vi "Next.vi"(7 "Address":string, 8 "Error In":errorcluster) -> (0 "Error Out":errorcluster)   [LabVIEW 2018, in "Tests.lvlib" / "Known Hosts.lvlib"]
uses:
  Known Hosts.lvlib
  src/Toolkit/Known Hosts/Type Definitions/Get Results.ctl
  <vilib>/Utility/error.llb/Clear Errors.vi
  src/Toolkit/Known Hosts/Support/Create from Session.vi
  <vilib>/Utility/sysdir.llb/Get System Directory.vi
  src/Toolkit/Known Host/Support/Create from Known Hosts.vi
  src/Toolkit/Known Host/Support/Destroy to Known Hosts.vi
  src/Toolkit/Known Hosts/Support/Destroy to Session.vi
  <vilib>/addons/_JKI Toolkits/Caraya/classes/Test/Test.lvclass
  <vilib>/addons/_JKI Toolkits/Caraya/classes/Assert/Assert.lvclass
  src/Toolkit/Known Hosts/Known Hosts.lvclass
  Tests.lvlib
  src/Toolkit/Session/Session.lvclass
  src/Toolkit/Known Host/Known Host.lvclass
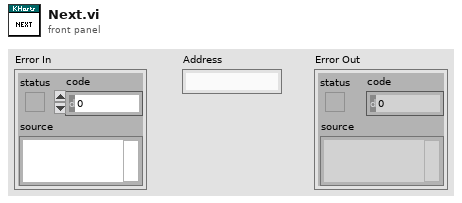
[diagram p1: front panel]
types:
  T1 = typedef "Toolkit.lvlib/Known Hosts.lvclass/Get Results.ctl" = i32
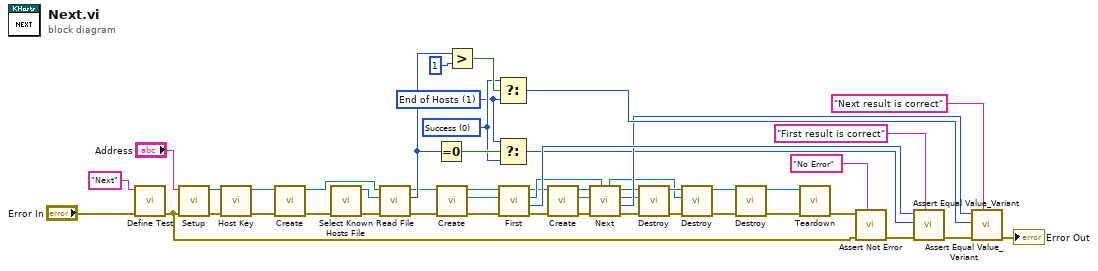
[diagram p0: block diagram]
diagram:
  w21 = T1 1 items=["Success", "End of Hosts"] ("Get Result")
  w22 = T1 0 items=["Success", "End of Hosts"] ("Get Result")
  n1 = call <vilib>:"Define Test.vi"("error in (no error)"="Error In", "Label (VI Title)"="Next") -> ("error out"=w41:errorcluster)  [unwired: 9 in]
  n2 = call "Setup.vi"("Error In"=w41, "Address In"="Address") -> ("Error Out"=w42:errorcluster, "Sesssion"=w43:refnum<class "Session.lvclass">)  [unwired: 7 in, 1 out]
  n3 = call "Host Key.vi"("Error In"=w42, "Session In"=w43) -> ("Error Out"=w1:errorcluster, "Sesssion Out"=w4:refnum<class "Session.lvclass">)  [unwired: 6 in, 2 out]
  n4 = call-poly "Create.vi"("Error In"=w1, "Session"=w4) -> ("Error Out"=w2:errorcluster, "Known Hosts"=w3:refnum<class "Known Hosts.lvclass">)  [unwired: 8 in]
  n5 = call "Select Known Hosts File.vi"("Error In"=w2) -> ("Error Out"=w47:errorcluster, "Known Hosts File"=w46:path)  [unwired: 9 in]
  n6 = call "Read File.vi"("Error In"=w47, "File"=w46, "Known Hosts In"=w3) -> ("Error Out"=w38:errorcluster, "Count"=w25:u64, "Known Hosts Out"=w20:refnum<class "Known Hosts.lvclass">)  [unwired: 6 in]
  n7 = Equal To 0?(x=w25) -> (x = 0?=w24:bool)
  n8 = call-poly "Create.vi"("Error In"=w38, "Known Hosts In"=w20) -> ("Error Out"=w37:errorcluster, "Known Host"=w17:refnum<class "Known Host.lvclass">, "Known Hosts Out"=w18:refnum<class "Known Hosts.lvclass">)  [unwired: 7 in]
  n9 = Greater?(x=w25, y=u64 1) -> (0:w26:bool)
  n10 = Select(t=w22, s=w26, f=w21) -> (s? t:f=w29:T1)
  n11 = Select(t=w21, s=w24, f=w22) -> (s? t:f=w23:T1)
  n12 = call "First.vi"("Error In"=w37, "Known Host In"=w17, "Known Hosts In"=w18) -> ("Error Out"=w34:errorcluster, "Result"=w36:T1, "Known Host Out"=w35:refnum<class "Known Host.lvclass">, "Known Hosts Out"=w19:refnum<class "Known Hosts.lvclass">)  [unwired: 5 in]
  n13 = call-poly "Create.vi"("Error In"=w34, "Known Hosts In"=w19) -> ("Error Out"=w33:errorcluster, "Known Host"=w15:refnum<class "Known Host.lvclass">, "Known Hosts Out"=w16:refnum<class "Known Hosts.lvclass">)  [unwired: 7 in]
  n14 = call "Next.vi"("Previous In"=w35, "Error In"=w33, "Next In"=w15, "Known Hosts In"=w16) -> ("Error Out"=w14:errorcluster, "Result"=w28:T1, "Next Out"=w12:refnum<class "Known Host.lvclass">, "Known Hosts Out"=w13:refnum<class "Known Hosts.lvclass">, "Previous Out"=w10:refnum<class "Known Host.lvclass">)  [unwired: 3 in]
  n15 = call-poly "Destroy.vi"("Error In"=w14, "Known Host"=w12, "KnownHosts In"=w13) -> ("Error Out"=w9:errorcluster, "KnownHosts Out"=w11:refnum<class "Known Hosts.lvclass">)  [unwired: 7 in]
  n16 = call-poly "Destroy.vi"("Error In"=w9, "Known Host"=w10, "KnownHosts In"=w11) -> ("Error Out"=w7:errorcluster, "KnownHosts Out"=w8:refnum<class "Known Hosts.lvclass">)  [unwired: 7 in]
  n17 = call-poly "Destroy.vi"("Error In"=w7, "Known Hosts"=w8) -> ("Error Out"=w6:errorcluster, "Session"=w5:refnum<class "Session.lvclass">)  [unwired: 8 in]
  n18 = call "Teardown.vi"("Error In"=w6, "Session"=w5) -> ("Error Out"=w39:errorcluster)  [unwired: 9 in]
  n19 = call <vilib>:"Assert Not Error.vi"("Label"="No Error", "error in (no error)"=w41, "Not Error?"=w39) -> ("error out"=w45:errorcluster)  [unwired: 8 in]
  n20 = call <vilib>:"Assert Equal Value_Variant.vi"("Label"="First result is correct", "error in (no error)"=w45, "Y"=w23, "X"=w36) -> ("error out"=w32:errorcluster)  [unwired: 7 in]
  n21 = call <vilib>:"Assert Equal Value_Variant.vi"("Label"="Next result is correct", "error in (no error)"=w32, "Y"=w29, "X"=w28) -> ("error out"=→"Error Out":errorcluster)  [unwired: 7 in]
